vi "CH_LM Config Display Smoothing Size Pulse.vi"(0 "Meter Index":i32, 2 "Number of Pulses (0:Auto)":i32, 5 "error in (no error)":errorcluster, 7 "Timeout / ms (3000)":i32=3000, 8 "Action (query)":bool, 9 "Lock Timeout / ms (1000)":i32=1000) -> (11 "Lock timed out":bool, 14 "Meter Index":i32, 16 "Number of Pulses":i32, 19 "error out":errorcluster)   [LabVIEW 2012, in "CH_LM.lvlib"]
doc: "Display data smoothing is controlled differently depending on the type of probe attached.\n\nThis command will set/query the display data smoothing window size expressed in number of pulses. \n\n<B>Attention:</B> This command will apply only when a pyroelectric probe is attached. Display data smoothing is not active in Joules mode when a thermopile probe is attached."
uses:
  CH_LM.lvlib
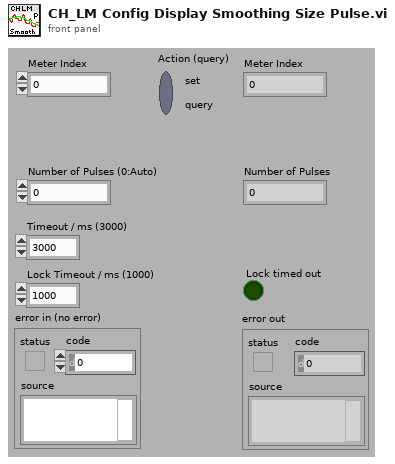
[diagram p1: front panel]
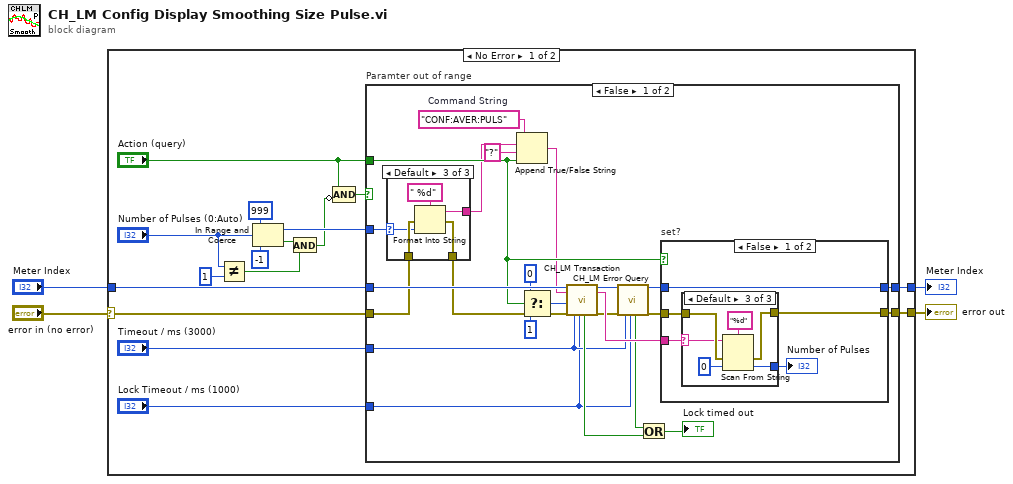
[diagram p0: block diagram]
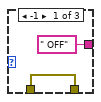
[diagram p2: hidden frame]
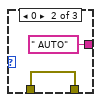
[diagram p3: hidden frame]
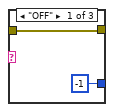
[diagram p4: hidden frame]
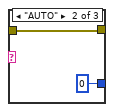
[diagram p5: hidden frame]
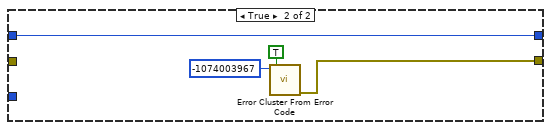
[diagram p7: hidden frame]
diagram:
  n1 = case shown="No Error" "error in (no error)" {
    selector: "error in (no error)" -> [w20 w76]
    tunnel: [w18 w76] -> w4
    tunnel: "Meter Index" -> [w19 w75]
    tunnel: [w17 w75] -> w1
    frame No Error {
      n2 = Not Equal?(x="Number of Pulses (0:Auto)", y=1) -> (x != y?=w7:bool)
      n3 = In Range and Coerce(upper limit=999, x="Number of Pulses (0:Auto)", lower limit=-1) -> (coerced(x)=w14:i32, In Range?=w6:bool)
      n4 = And(x=w6, y=w7) -> (x .and. y?=w5:bool)
      n5 = Compound Arithmetic op=AND("Action (query)", invert w5) -> (w10:bool)
      n6 = case "Paramter out of range" shown="False" w10 {
        tunnel: w20 -> [w25 _]
        tunnel: w19 -> [w44 w74]
        tunnel: [w41 w72] -> w18
        tunnel: [w36 w74] -> w17
        tunnel: "Timeout / ms (3000)" -> [w28 _]
        tunnel: "Lock Timeout / ms (1000)" -> [w27 _]
        tunnel: w14 -> [w21 _]
        tunnel: "Action (query)" -> [w26 _]
        frame False {
          w43 = "CONF:AVER:PULS"  # Command String
          n7 = case shown="Default" w21 {
            selector: w21 -> [_ _ w49]
            tunnel: w25 -> [w45 w48 w52]
            tunnel: [w45 w48 w51] -> w24
            tunnel: [" OFF" " AUTO" w50] -> w22
            frame -1 {
            }
            frame 0 {
            }
            frame Default {
              n8 = Format Into String(format string=" %d", error in=w52, w49) -> (resulting string=w50:string, error out=w51:errorcluster)  [unwired: 1 in]
            }
          }
          n9 = Append True/False String(1:w26, 2:"?" ("true string"), 3:w22, 4:w43) -> (0:w23:string)
          n10 = Select(t=0, s=w26, f=1 ("NofStrings (-1:all)")) -> (s? t:f=w38:i32)
          n11 = call "CH_LM Transaction.vi"("Meter Index"=w44, "Command String"=w23, "NofStrings (-1:all)"=w38, "error in (no error)"=w24, "Timeout / ms (3000)"=w28, "Lock Timeout / ms (1000)"=w27) -> ("Lock timed out"=w30:bool, "Meter Index"=w35:i32, "Response"=w42:string, "error out"=w33:errorcluster)  [unwired: 10 out]
          n12 = call "CH_LM Error Query.vi"("Meter Index"=w35, "error in (no error)"=w33, "Timeout / ms (3000)"=w28, "Lock Timeout / ms (1000)"=w27) -> ("Lock timed out"=w31:bool, "Meter Index"=w34:i32, "error out"=w32:errorcluster)  [unwired: 13 out]
          n13 = Or(x=w31, y=w30) -> (x .or. y?=→"Lock timed out":bool)
          n14 = case "set?" shown="False" w26 {
            tunnel: w42 -> [w54 _]
            tunnel: w32 -> [w58 w70]
            tunnel: [w57 w70] -> w41
            tunnel: w34 -> [w56 w69]
            tunnel: [w56 w69] -> w36
            frame False {
              n15 = case shown="Default" w54 {
                selector: w54 -> [_ _ w63]
                tunnel: w58 -> [w59 w62 w68]
                tunnel: [w59 w62 w67] -> w57
                tunnel: [-1 ("default value 1") 0 ("default value 1") w64] -> w55
                frame "OFF" {
                }
                frame "AUTO" {
                }
                frame Default {
                  n16 = Scan From String(format string="%d", input string=w63, error in=w68, default 1=0 ("default value 1")) -> (error out=w67:errorcluster, output 1=w64:i32)  [unwired: 1 in, 2 out]
                }
              }
              "Number of Pulses" <- w55
            }
            frame True {
            }
          }
        }
        frame True {
          n17 = call <vilib>:"Error Cluster From Error Code.vi"("show call chain? (False)"=TRUE, "error code (0)"=-1074003967) -> ("error out"=w72:errorcluster)  [unwired: 1 in, 6 out]
        }
      }
    }
    frame Error {
    }
  }
  "error out" <- w4
  "Meter Index" <- w1
